vi "Identify.vi"(8 "error in (no error)":errorcluster, 11 "File Parsing Interface in":refnum<class "File Parsing Interface.lvclass">) -> (0 "error out":errorcluster, 2 "Plugin is Valid":bool, 3 "File Parsing Interface out":refnum<class "File Parsing Interface.lvclass">)   [LabVIEW 2018, in "File Parsing Interface.lvlib" / "File Parsing Interface.lvclass"]
uses:
  File Parsing Interface.lvclass
  Plugins/FPF.lvlibp/Factory Plugin Framework.lvclass
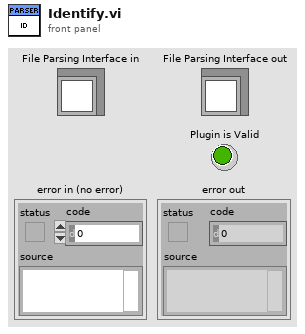
[diagram p1: front panel]
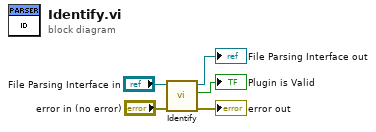
[diagram p0: block diagram]
diagram:
  n1 = call-parent "Identify.vi"("error in (no error)"="error in (no error)", "Factory Plugin Framework in"="File Parsing Interface in") -> ("error out"=→"error out":errorcluster, "Plugin is Valid"=→"Plugin is Valid":bool, "Factory Plugin Framework out"=→"File Parsing Interface out":refnum<class "File Parsing Interface.lvclass">)  [unwired: 7 in]
